vi "Close TDMS.vi"(8 "error in (no error)":errorcluster, 11 "Devantech SRF05 in":refnum<class "Devantech SRF05.lvclass">) -> (0 "error out":errorcluster, 3 "Devantech SRF05 out":refnum<class "Devantech SRF05.lvclass">)   [LabVIEW 2019, in "Devantech SRF05.lvclass"]
doc: "Closes the tdms file."
uses:
  Devantech SRF05.lvclass
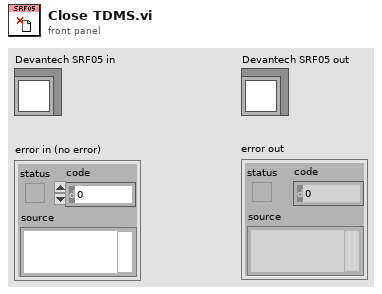
[diagram p1: front panel]
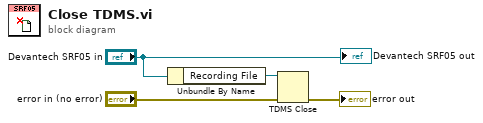
[diagram p0: block diagram]
diagram:
  n1 = Unbundle By Name("Devantech SRF05 in") -> ("Recording File"=w2:refnum<k34>)
  n2 = TDMS Close(8:"error in (no error)", 11:w2) -> (0:→"error out":errorcluster)  [unwired: 1 out]
  "Devantech SRF05 out" <- "Devantech SRF05 in"
